vi "Reg Key Constants.vi"() -> (0 "Default Templates Folder":path, 1 "String Value Name":string, 2 "Subkey Path":string, 3 "Root Key":T1=enum."HKEY_CURRENT_USER")   [LabVIEW 2021]
doc: "<add documentation here>"
uses:
  <vilib>/registry/registry.llb/Registry RtKey.ctl
  <vilib>/Utility/sysdir.llb/System Directory Type.ctl
panel:
  # "Development\nControls or indicators that are useful for development or testing, but which are not outputs of the VI."
  # "Input\nInputs to the VI"
  # "Output\nOutputs of the VI"
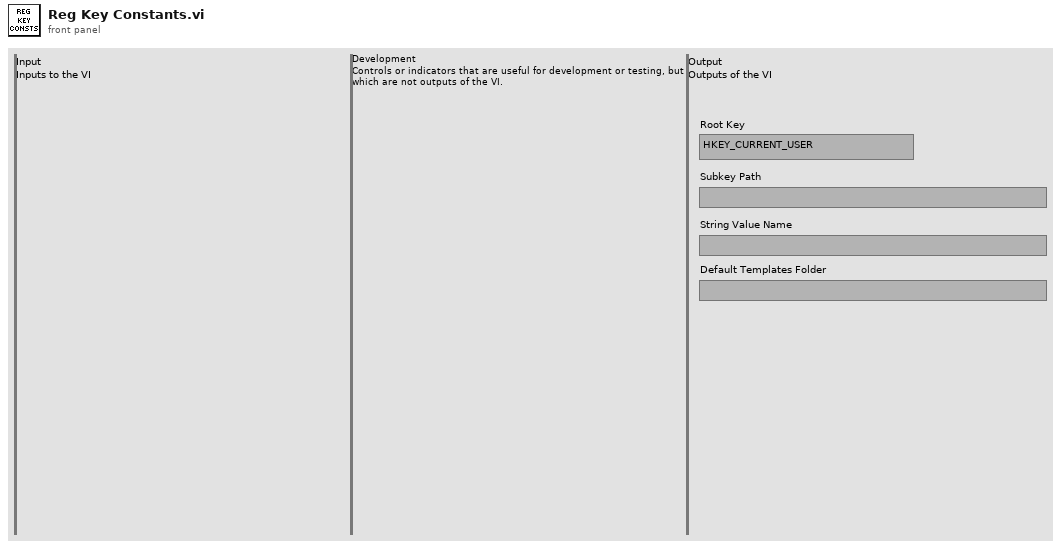
[diagram p1: front panel]
types:
  T1 = typedef "Registry RtKey.ctl" = enum32{"HKEY_CLASSES_ROOT", "HKEY_CURRENT_USER", "HKEY_LOCAL_MACHINE", "HKEY_USERS", "HKEY_PERFORMANCE_DATA", "HKEY_CURRENT_CONFIG", "HKEY_DYN_DATA"}
  T2 = typedef "System Directory Type.ctl" = i32
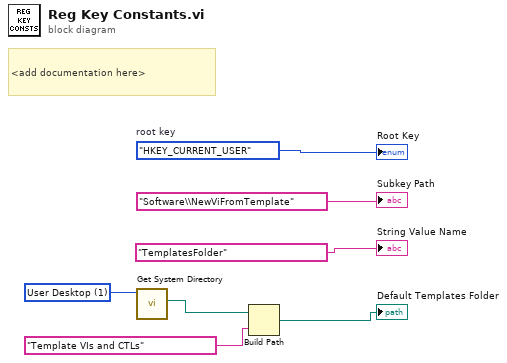
[diagram p0: block diagram]
diagram:
  w4 = T2 1 items=["User Home"=0, "User Desktop"=1, "User Documents"=2, "User Application Data"=3, "User Preferences"=4, "User Temporary"=5, "Public Documents"=6, "Public Application Data"=7, "Public Preferences"=8, "Public Cache"=13, "System Core Libraries"=9, "System Installed Libraries"=10, "Application Files"=11, "Boot Volume Root"=12] ("system directory type")
  w5 = Registry_RtKey."HKEY_CURRENT_USER"  # root key
  # "<add documentation here>"
  n1 = call <vilib>:"Get System Directory.vi"("system directory type"=w4) -> ("system directory"=w3:path)  [unwired: 10 in]
  n2 = Build Path(base path=w3, name or relative path="Template VIs and CTLs") -> (appended path=→"Default Templates Folder":path)
  "Subkey Path" <- "Software\\NewViFromTemplate"
  "String Value Name" <- "TemplatesFolder"
  "Root Key" <- w5
